vi "程序设置-保存注释.vi"(8 "error in":errorcluster caption="错误输入（无错误）", 10 "程序注释":string, 11 "程序号":i32) -> (0 "error out":errorcluster)   [LabVIEW 2017]
uses:
  <vilib>/Utility/xml.llb/Write to XML File(string).vi
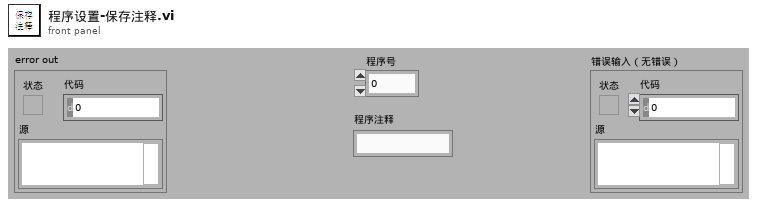
[diagram p1: front panel]
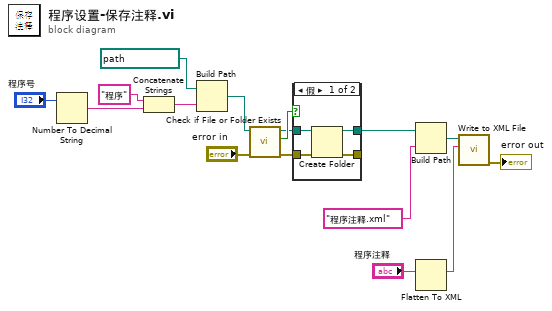
[diagram p0: block diagram]
diagram:
  n1 = Number To Decimal String(number="程序号") -> (decimal integer string=w8:string)  [unwired: 1 in]
  n2 = Concatenate Strings("程序" ("字符串"), w8) -> (w11:string)
  n3 = Build Path(base path=path "D:/程序参数" ("基路径"), name or relative path=w11) -> (appended path=w7:path)
  n4 = call <vilib>:"Check if File or Folder Exists.vi"("error in (no error)"="error in", "path"=w7) -> ("error out"=w4:errorcluster, "file or folder exists?"=w6:bool, "dup path"=w5:path)  [unwired: 7 in]
  n5 = case shown="假" w6 {
    tunnel: w5 -> [w20 w22]
    tunnel: w4 -> [w19 w21]
    tunnel: [w18 w22] -> w3
    tunnel: [w17 w21] -> _
    frame False {
      n6 = Create Folder(path (use dialog)=w20, error in=w19) -> (created path=w18:path, error out=w17:errorcluster)  [unwired: 1 in, 1 out]
    }
    frame True {
    }
  }
  n7 = Build Path(base path=w3, name or relative path="程序注释.xml" ("名称或相对路径")) -> (appended path=w14:path)
  n8 = Flatten To XML(anything="程序注释") -> (xml string=w13:string)
  n9 = call-poly <vilib>:"Write to XML File.vi"("XML Input"=w13, "XML File Path"=w14) -> ("error out"=→"error out":errorcluster)  [unwired: 7 in, 2 out]
